vi "midiOutPlayer.Launch.vi"(8 "error in":errorcluster, 10 "file events":refnum<class "midi-file-event.lvclass">[](array[class]), 11 "midiPlayer in":refnum<class "midiPlayer.lvclass">) -> (0 "error out":errorcluster, 3 "midiPlayer out":refnum<class "midiPlayer.lvclass">)   [LabVIEW 2020, in "midiPlayer.lvclass"]
uses:
  midiPlayer.lvclass
  midiPlayer.lvclass/midiPlayer.ctl
  midiOutPlayer.Core.vi
  midi-file-events/midi-file-event.lvclass
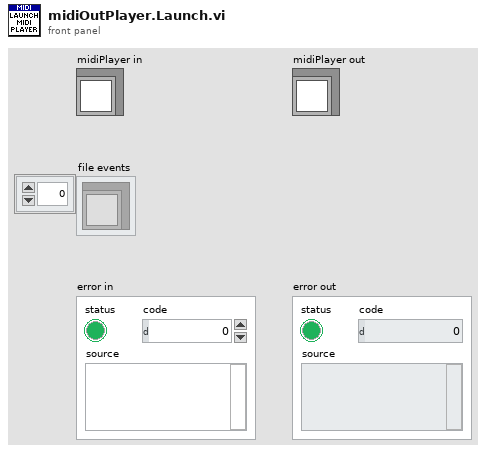
[diagram p1: front panel]
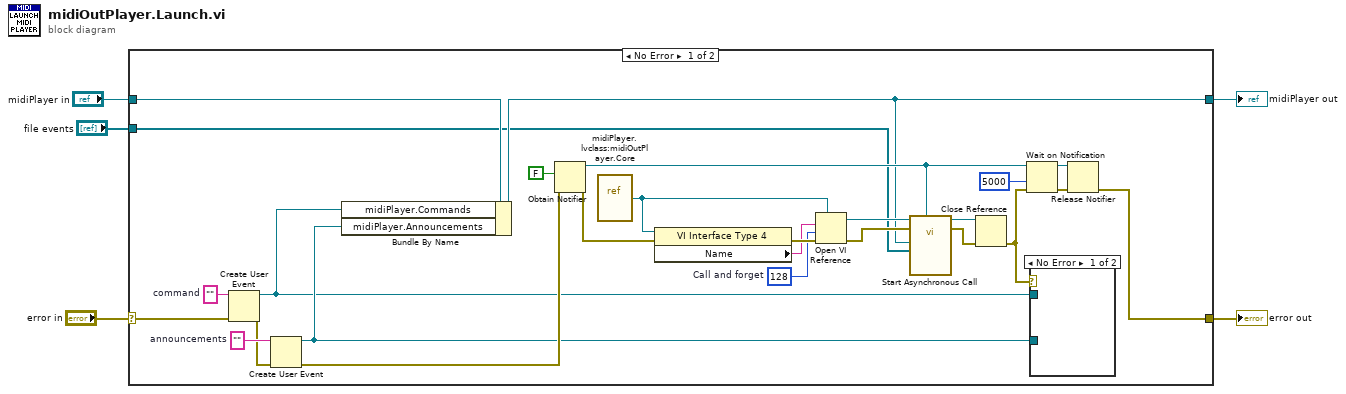
[diagram p0: block diagram]
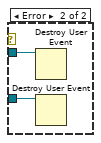
[diagram p2: hidden frame]
diagram:
  n1 = case shown="No Error" "error in" {
    selector: "error in" -> [w23 w35]
    tunnel: [w8 w35] -> w4
    tunnel: "midiPlayer in" -> [w11 w34]
    tunnel: "file events" -> [w6 _]
    tunnel: [w7 w34] -> w2
    frame No Error {
      w19 = ""  # announcements
      w22 = 128  # Call and forget
      w31 = ""  # command
      n2 = Create User Event(user event datatype=w31, error in=w23) -> (user event=w9:refnum<user-event>, error out=w18:errorcluster)
      n3 = Create User Event(user event datatype=w19, error in=w18) -> (user event=w10:refnum<user-event>, error out=w17:errorcluster)
      n4 = Bundle By Name(cluster=w11, "midiPlayer.Commands"=w9, "midiPlayer.Announcements"=w10) -> (w7:refnum<class "midiPlayer.lvclass">)
      n5 = Obtain Notifier(notification data type=FALSE, error in (no error)=w17) -> (notifier out=w16:refnum<notifier>, error out=w24:errorcluster)  [unwired: 2 in, 1 out]
      n6 = vi-ref "midiPlayer.lvclass:midiOutPlayer.Core.vi"() -> (w27:refnum<vi>)
      n7 = property class="VI Interface Type 4"(reference=w27, error in=w24) -> (error out=w26:errorcluster, "Name"=w25:string)  [unwired: 1 out]
      n8 = Open VI Reference(type specifier VI Refnum (for type only)=w27, vi path=w25, options=w22, error in (no error)=w26) -> (vi reference=w28:refnum<vi>, error out=w29:errorcluster)  [unwired: 2 in]
      n9 = call-by-ref "Start Asynchronous Call"(reference=w28, error in=w29, "notifier out"=w16, "file events"=w6, "midiPlayer"=w7) -> (reference out=w21:refnum<vi>, error out=w20:errorcluster)  [unwired: 9 in]
      n10 = Close Reference(reference=w21, error in (no error)=w20) -> (error out=w15:errorcluster)
      n11 = Wait on Notification(notifier=w16, timeout in ms (-1)=5000, error in (no error)=w15) -> (notifier out=w14:refnum<notifier>, error out=w13:errorcluster)  [unwired: 1 in, 2 out]
      n12 = case shown="No Error" w15 {
        tunnel: w9 -> [_ w33]
        tunnel: w10 -> [_ w32]
        frame No Error {
        }
        frame Error {
          n13 = Destroy User Event(user event=w33) -> ()  [unwired: 1 in, 1 out]
          n14 = Destroy User Event(user event=w32) -> ()  [unwired: 1 in, 1 out]
        }
      }
      n15 = Release Notifier(notifier=w14, error in (no error)=w13) -> (error out=w8:errorcluster)  [unwired: 1 in, 2 out]
    }
    frame Error {
    }
  }
  "error out" <- w4
  "midiPlayer out" <- w2
